vi "Solve2.vi"(8 "Error In":errorcluster, 11 "object in":refnum<class "2021_12.lvclass">) -> (0 "Error Out":errorcluster, 2 "Result":u64, 3 "object out":refnum<class "2021_12.lvclass">)   [LabVIEW 2020, in "2021_12.lvclass"]
uses:
  2021_12.lvclass
  12_Cave_class/12_Cave.lvclass
  2021_12.lvclass/2021_12.ctl
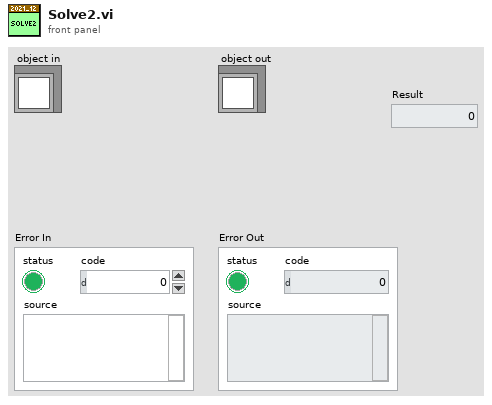
[diagram p1: front panel]
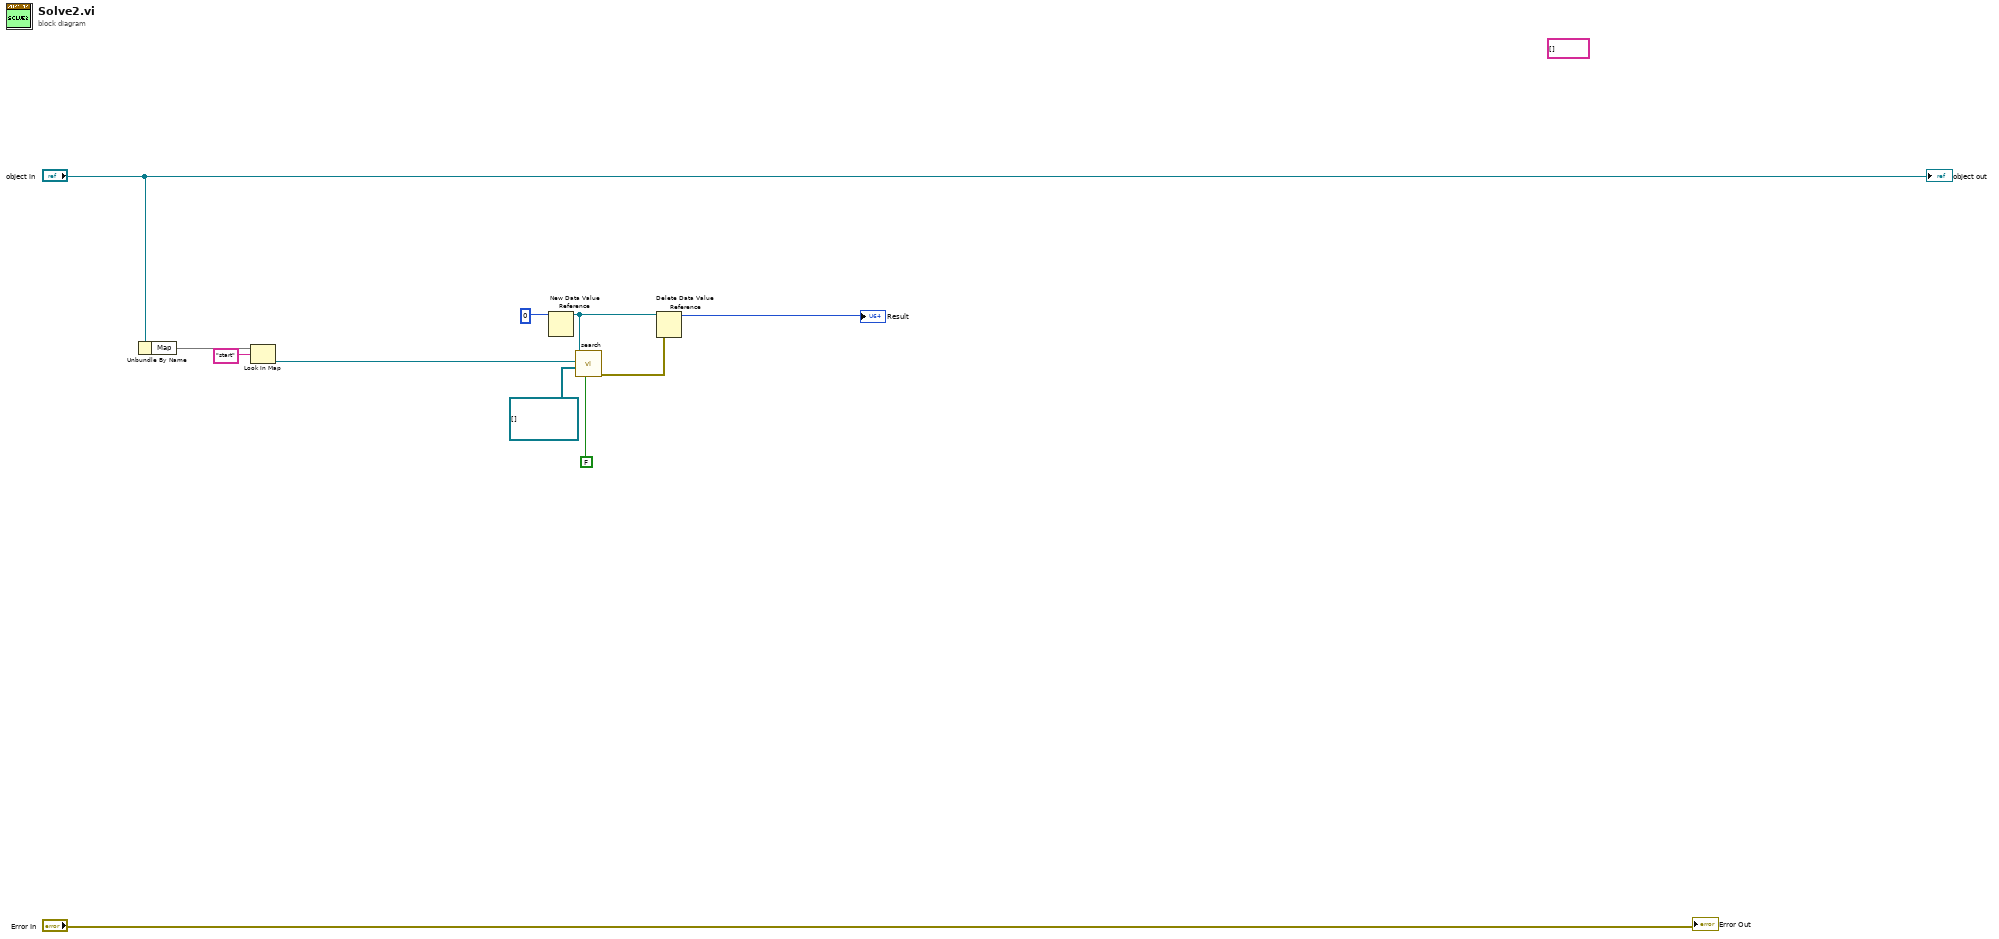
[diagram p0: block diagram]
diagram:
  (unwired) string[] [] ("LinesOfCode")
  n1 = Unbundle By Name("object in") -> ("Map"=w9:map{string, refnum<class "12_Cave.lvclass">})
  n2 = Look In Map(map=w9, key="start" ("y")) -> (value=w5:refnum<class "12_Cave.lvclass">)  [unwired: 1 in, 1 out]
  n3 = New Data Value Reference(data value=0) -> (data value reference=w2:refnum<data-value>)  [unwired: 1 in, 1 out]
  n4 = call "search.vi"("Small Cave Visited Twize"=FALSE, "Path(Nodes)"=refnum<class "12_Cave.lvclass">[] [] ("PathIn"), "FronNode"=w5, "NoOfPath"=w2) -> ("Error Out"=w6:errorcluster)  [unwired: 6 in, 1 out]
  n5 = Delete Data Value Reference(data value reference=w2, error in=w6) -> (data value=→"Result":i32)  [unwired: 1 out]
  "Error Out" <- "Error In"
  "object out" <- "object in"
